vi "Position_speed.vi"(0 "Px":dbl, 5 "Py":dbl, 7 "Vx":dbl, 9 "Vy":dbl, 11 "Delta_T":dbl, 12 "F":dbl, 13 "f":dbl, 14 "m":dbl, 15 "Theta":dbl) -> (4 "Px":dbl, 6 "Py":dbl, 8 "Vx":dbl, 10 "Vy":dbl)   [LabVIEW 2015]
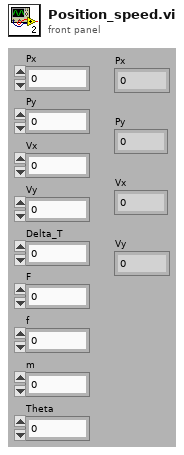
[diagram p1: front panel]
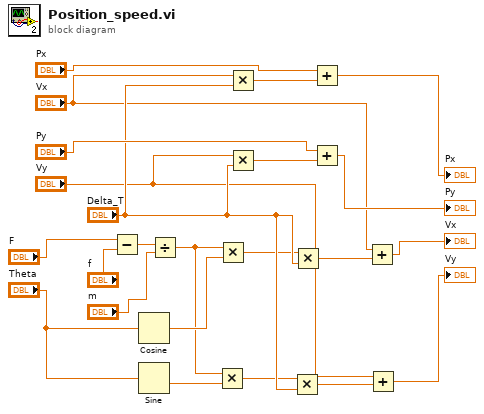
[diagram p0: block diagram]
diagram:
  n1 = Subtract(x="F", y="f") -> (x-y=w2:dbl)
  n2 = Cosine(x="Theta") -> (cos(x)=w8:dbl)
  n3 = Sine(x="Theta") -> (sin(x)=w9:dbl)
  n4 = Divide(x=w2, y="m") -> (x/y=w1:dbl)
  n5 = Multiply(x=w1, y=w9) -> (x*y=w7:dbl)
  n6 = Multiply(x=w1, y=w8) -> (x*y=w3:dbl)
  n7 = Multiply(x="Vx", y="Delta_T") -> (x*y=w15:dbl)
  n8 = Multiply(x="Vy", y="Delta_T") -> (x*y=w16:dbl)
  n9 = Multiply(x=w7, y="Delta_T") -> (x*y=w12:dbl)
  n10 = Multiply(x=w3, y="Delta_T") -> (x*y=w11:dbl)
  n11 = Add(x="Px", y=w15) -> (x+y=→"Px":dbl)
  n12 = Add(x="Py", y=w16) -> (x+y=→"Py":dbl)
  n13 = Add(x="Vx", y=w11) -> (x+y=→"Vx":dbl)
  n14 = Add(x="Vy", y=w12) -> (x+y=→"Vy":dbl)
